vi "RichToFlatni_measurementlink_sessionmanagement_v1_SessionInformation.vi"(5 "OutputClusterType":T1, 11 "InputCluster":T4) -> (3 "OutputCluster":T1)   [LabVIEW 2024, in "ni.measurementlink.sessionmanagement.v1.api.lvlib"]
uses:
  ni.measurementlink.sessionmanagement.v1.api.lvlib
  ni_measurementlink_sessionmanagement_v1_SessionInformation.ctl
  nidevice_grpc_Session.ctl
  ni_measurementlink_sessionmanagement_v1_ChannelMapping.ctl
  ni_measurementlink_sessionmanagement_v1_SessionInformation_Flat.ctl
  nidevice_grpc_Session_Flat.ctl
  ni_measurementlink_sessionmanagement_v1_ChannelMapping_Flat.ctl
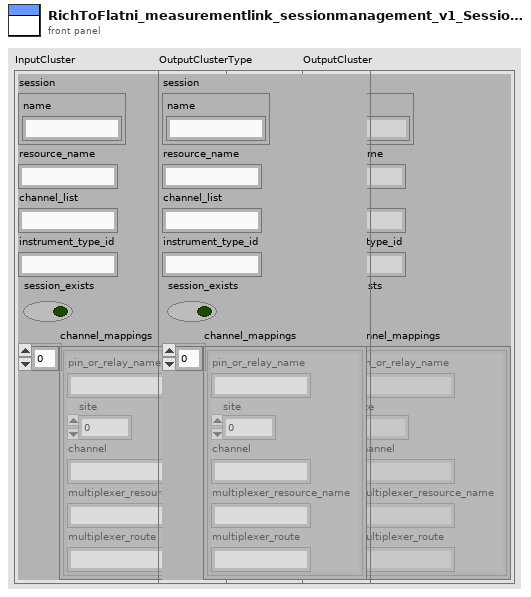
[diagram p1: front panel]
types:
  T1 = typedef "ni.measurementlink.sessionmanagement.v1.api.lvlib/ni_measurementlink_sessionmanagement_v1_SessionInformation_Flat.ctl" = cluster{"session":T2, "resource_name":string, "channel_list":string, "instrument_type_id":string, "session_exists":bool, "channel_mappings":T3[]}
  T2 = typedef "ni.measurementlink.sessionmanagement.v1.api.lvlib/nidevice_grpc_Session_Flat.ctl" = cluster{"name":string}
  T3 = typedef "ni.measurementlink.sessionmanagement.v1.api.lvlib/ni_measurementlink_sessionmanagement_v1_ChannelMapping_Flat.ctl" = cluster{"pin_or_relay_name":string, "site":i32, "channel":string, "multiplexer_resource_name":string, "multiplexer_route":string}
  T4 = typedef "ni.measurementlink.sessionmanagement.v1.api.lvlib/ni_measurementlink_sessionmanagement_v1_SessionInformation.ctl" = cluster{"session":T5, "resource_name":string, "channel_list":string, "instrument_type_id":string, "session_exists":bool, "channel_mappings":T6[]}
  T5 = typedef "ni.measurementlink.sessionmanagement.v1.api.lvlib/nidevice_grpc_Session.ctl" = cluster{"name":string}
  T6 = typedef "ni.measurementlink.sessionmanagement.v1.api.lvlib/ni_measurementlink_sessionmanagement_v1_ChannelMapping.ctl" = cluster{"pin_or_relay_name":string, "site":i32, "channel":string, "multiplexer_resource_name":string, "multiplexer_route":string}
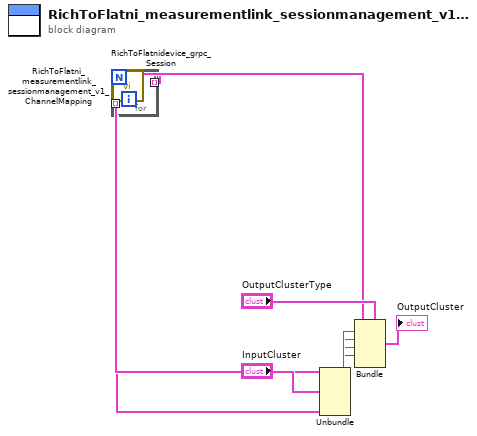
[diagram p0: block diagram]
diagram:
  n1 = Unbundle "Unbundle"("InputCluster") -> ("session"=w8:T5, "resource_name"=w6:string, "channel_list"=w5:string, "instrument_type_id"=w4:string, "session_exists"=w3:bool, "channel_mappings"=w2:T6[])
  n2 = for {
    tunnel: w2 -> [w13] mode=indexing
    tunnel: [w12] -> w1 mode=indexing
    n3 = call "RichToFlatni_measurementlink_sessionmanagement_v1_ChannelMapping.vi"("InputCluster"=w13) -> ("OutputCluster"=w12:T3)  [unwired: 10 in]
  }
  n4 = call "RichToFlatnidevice_grpc_Session.vi"("InputCluster"=w8) -> ("OutputCluster"=w7:T2)  [unwired: 10 in]
  n5 = Bundle "Bundle"(cluster="OutputClusterType", "session"=w7, "resource_name"=w6, "channel_list"=w5, "instrument_type_id"=w4, "session_exists"=w3, "channel_mappings"=w1) -> (→"OutputCluster":T1)
